vi "array_Global 2.vi"() -> ()   [LabVIEW 2014]
panel:
  in  "Array Defined":dbl[][](array[numeric])=[[5.0, 10.0, 15.0], [0.0, 20.0, 25.0], [5.0, 0.0, 10.0], [10.0, 20.0, 30.0], [5.0, 10.0, 0.0]]
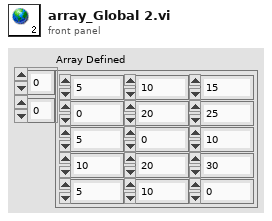
[diagram p1: front panel]
diagram:
